vi "svx_Data to Process (DAQmx).vi"(0 "acquisition task":T1={"AI device settings"={"AI DAQmx TaskID"="", "response"=[{"AI physical channel"="Dev1/ai0", "AI channel settings"={"max value [V]"=10.0, "min value [V]"=-10.0, "terminal config"=10083, "DSA channel settings"={"coupling"=10045, "enable IEPE excitation"=FALSE, "IEPE current [mA]"=4.0}}}]}, "acquisition type"=enum."Finite", "measurement settings"={"AI sampling frequency"=51200.0, "AO sampling frequency"=51200.0, "AI block size"=0, "AO block Size"=0, "block duration [ms]"=100.0, "number of AI channels"=0, "device propagation delay [samples]"=0.0, "DUT propagation time [s]"=0.0}, "settling settings"={"settle time"=0.015599999576807022, "settle cycles"=5}, "integration settings"={"integration time"=0.015599999576807022, "integration cycles"=5}, "AO device settings"={"AO DAQmx taskID"="", "excitation"=[]}, "acquisition accounting"={"initial read size [samples]"=0, "read offset [samples]"=0, "read length [samples]"=0, "blocks to settle [samples]"=0, "min delay until transition [samples]"=0}, "frequency range"={"start frequency"=-1.0, "stop frequency"=-1.0}, "block type"=enum."Initialize", "source settings"={"signal type"=enum."Sine wave", "frequency"=0.0, "total amplitude"=0.0, "frequencies"=[1.0], "relative amplitudes"=[1.0], "offset"=1.0, "total amplitude list"=[1.0], "ramping rate"=0.0}, "chirp settings"={"amplitude"=0.0, "frequency range"={"start (Hz)"=20.0, "stop (Hz)"=20000.0, "frequency spacing"=enum."Logarithmic"}, "sampling info"={"Fs"=50000.0, "chirp duration [s]"=3.0}, "initial states"={"frequency [Hz]"=20.0, "phase [rad]"=0.0, "elapsed time [s]"=0.0}, "frequency slope"=0.0, "maximum harmonic"=0, "prefix len [samples]"={"integer"=0, "fractional"=0.0}}} {"chirp settings"."frequency slope" format="%.2f"; "chirp settings"."prefix len [samples]"."fractional" format="%.2p"; "chirp settings"."initial states"."elapsed time [s]" format="%.2f"; "chirp settings"."initial states"."phase [rad]" format="%.2f"; "chirp settings"."initial states"."frequency [Hz]" format="%.2f"; "chirp settings"."sampling info"."chirp duration [s]" format="%.2f"; "chirp settings"."sampling info"."Fs" format="%.2p"; "chirp settings"."frequency range"."stop (Hz)" format="%.2f"; "chirp settings"."frequency range"."start (Hz)" format="%.2f"; "chirp settings"."amplitude" format="%.2f"; "source settings"."total amplitude" format="%.2f"; "source settings"."relative amplitudes" format="%.2f"; "source settings"."frequencies" format="%.2f"; "source settings"."total amplitude list" format="%.2f"; "source settings"."ramping rate" format="%.4f"; "source settings"."offset" format="%.2f"; "source settings"."frequency" format="%.2f"; "frequency range"."stop frequency" format="%.2f"; "frequency range"."start frequency" format="%.2f"; "AO device settings"."excitation"."AO channel settings"."terminal config" items=["Default"=-1, "Differential"=10106, "Pseudodifferential"=12529]; "AI device settings"."response"."AI channel settings"."DSA channel settings"."IEPE current [mA]" min=0.0 max=20.0 format="%.1f"; "AI device settings"."response"."AI channel settings"."DSA channel settings"."coupling" items=["AC"=10045, "DC"=10050, "GND"=10066]; "AI device settings"."response"."AI channel settings"."min value [V]" format="%.2f"; "AI device settings"."response"."AI channel settings"."terminal config" items=["Default"=-1, "RSE"=10083, "NRSE"=10078, "Differential"=10106, "Pseudodifferential"=12529]; "AI device settings"."response"."AI channel settings"."max value [V]" format="%.2f"; "integration settings"."integration time" format="%.2p"; "settling settings"."settle time" format="%.2p"; "measurement settings"."DUT propagation time [s]" format="%.2f"; "measurement settings"."AO sampling frequency" format="%.2f"; "measurement settings"."AI sampling frequency" format="%.2f"}, 5 "waveform data":waveform(dbl)[](array[waveform]), 11 "error in (no error)":errorcluster) -> (4 "acquisition task":T1={"AI device settings"={"AI DAQmx TaskID"="", "response"=[{"AI physical channel"="Dev1/ai0", "AI channel settings"={"max value [V]"=10.0, "min value [V]"=-10.0, "terminal config"=10083, "DSA channel settings"={"coupling"=10045, "enable IEPE excitation"=FALSE, "IEPE current [mA]"=4.0}}}]}, "acquisition type"=enum."Finite", "measurement settings"={"AI sampling frequency"=51200.0, "AO sampling frequency"=51200.0, "AI block size"=0, "AO block Size"=0, "block duration [ms]"=100.0, "number of AI channels"=0, "device propagation delay [samples]"=0.0, "DUT propagation time [s]"=0.0}, "settling settings"={"settle time"=0.015599999576807022, "settle cycles"=5}, "integration settings"={"integration time"=0.015599999576807022, "integration cycles"=5}, "AO device settings"={"AO DAQmx taskID"="", "excitation"=[]}, "acquisition accounting"={"initial read size [samples]"=0, "read offset [samples]"=0, "read length [samples]"=0, "blocks to settle [samples]"=0, "min delay until transition [samples]"=0}, "frequency range"={"start frequency"=-1.0, "stop frequency"=-1.0}, "block type"=enum."Initialize", "source settings"={"signal type"=enum."Sine wave", "frequency"=0.0, "total amplitude"=0.0, "frequencies"=[1.0], "relative amplitudes"=[1.0], "offset"=1.0, "total amplitude list"=[1.0], "ramping rate"=0.0}, "chirp settings"={"amplitude"=0.0, "frequency range"={"start (Hz)"=20.0, "stop (Hz)"=20000.0, "frequency spacing"=enum."Logarithmic"}, "sampling info"={"Fs"=50000.0, "chirp duration [s]"=3.0}, "initial states"={"frequency [Hz]"=20.0, "phase [rad]"=0.0, "elapsed time [s]"=0.0}, "frequency slope"=0.0, "maximum harmonic"=0, "prefix len [samples]"={"integer"=0, "fractional"=0.0}}} {"chirp settings"."frequency slope" format="%.2f"; "chirp settings"."prefix len [samples]"."fractional" format="%.2p"; "chirp settings"."initial states"."elapsed time [s]" format="%.2f"; "chirp settings"."initial states"."phase [rad]" format="%.2f"; "chirp settings"."initial states"."frequency [Hz]" format="%.2f"; "chirp settings"."sampling info"."chirp duration [s]" format="%.2f"; "chirp settings"."sampling info"."Fs" format="%.2p"; "chirp settings"."frequency range"."stop (Hz)" format="%.2f"; "chirp settings"."frequency range"."start (Hz)" format="%.2f"; "chirp settings"."amplitude" format="%.2f"; "source settings"."total amplitude" format="%.2f"; "source settings"."relative amplitudes" format="%.2f"; "source settings"."frequencies" format="%.2f"; "source settings"."total amplitude list" format="%.2f"; "source settings"."ramping rate" format="%.4f"; "source settings"."offset" format="%.2f"; "source settings"."frequency" format="%.2f"; "frequency range"."stop frequency" format="%.2f"; "frequency range"."start frequency" format="%.2f"; "AO device settings"."excitation"."AO channel settings"."terminal config" items=["Default"=-1, "Differential"=10106, "Pseudodifferential"=12529]; "AI device settings"."response"."AI channel settings"."DSA channel settings"."IEPE current [mA]" min=0.0 max=20.0 format="%.1f"; "AI device settings"."response"."AI channel settings"."DSA channel settings"."coupling" items=["AC"=10045, "DC"=10050, "GND"=10066]; "AI device settings"."response"."AI channel settings"."min value [V]" format="%.2f"; "AI device settings"."response"."AI channel settings"."terminal config" items=["Default"=-1, "RSE"=10083, "NRSE"=10078, "Differential"=10106, "Pseudodifferential"=12529]; "AI device settings"."response"."AI channel settings"."max value [V]" format="%.2f"; "integration settings"."integration time" format="%.2p"; "settling settings"."settle time" format="%.2p"; "measurement settings"."DUT propagation time [s]" format="%.2f"; "measurement settings"."AO sampling frequency" format="%.2f"; "measurement settings"."AI sampling frequency" format="%.2f"}, 6 "data to process":waveform(dbl)[](array[waveform]), 8 "new data to process":bool, 15 "error out":errorcluster)   [LabVIEW 2017]
uses:
  <vilib>/addons/Sound and Vibration/Example Support/Audio/DAQmx/svx_Acquisition Task (DAQmx).ctl
  <vilib>/addons/_NISVFA/_Shared subVIs/Controls/svc_Channel Settings.ctl
  <vilib>/addons/_NISVFA/_Shared subVIs/Controls/svc_DSA Channel Settings.ctl
  <vilib>/addons/_NISVFA/_Generation/subVIs/sv_Chirp Settings.ctl
  <vilib>/Waveform/WDTOps.llb/WDT Get Waveform Subset DBL (LV80).vi
  <vilib>/addons/_NISVFA/_Generation/SoundVib_Generation.lvlib
panel:
  in  "empty":waveform(dbl)[](array[waveform])
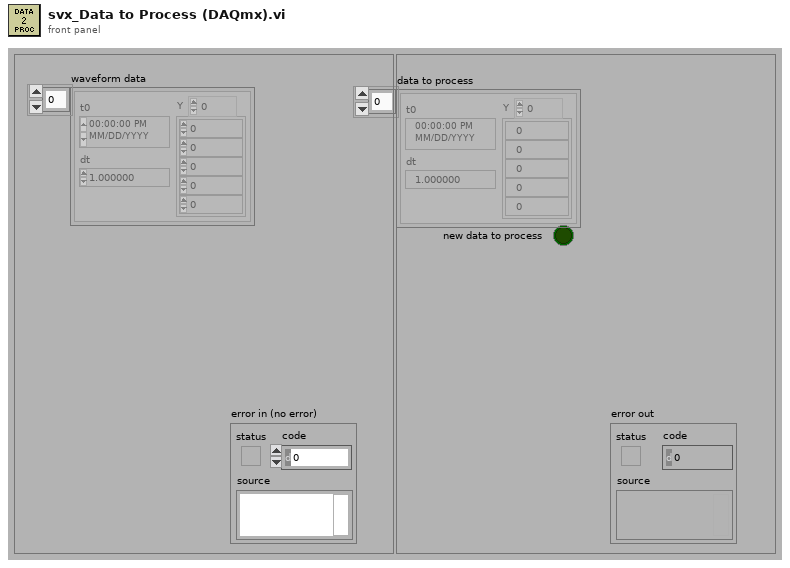
[diagram p1: front panel]
types:
  T1 = typedef "svx_Acquisition Task (DAQmx).ctl" = cluster{"AI device settings":cluster{"AI DAQmx TaskID":refnum<k21>, "response":cluster{"AI physical channel":tag, "AI channel settings":T2}[]}, "acquisition type":enum16{"Finite", "Averaged", "Settled", "Amplitude Sweep", "Stepped Frequency Sweep", "Continuous Frequency Sweep"}, "measurement settings":cluster{"AI sampling frequency":dbl, "AO sampling frequency":dbl, "AI block size":i32, "AO block Size":i32, "block duration [ms]":dbl, "number of AI channels":i32, "device propagation delay [samples]":dbl, "DUT propagation time [s]":dbl}, "settling settings":cluster{"settle time":dbl, "settle cycles":i32}, "integration settings":cluster{"integration time":dbl, "integration cycles":i32}, "AO device settings":cluster{"AO DAQmx taskID":refnum<k21>, "excitation":cluster{"AO physical channel":tag, "AO channel settings":cluster{"maximum value (10 V)":dbl, "minimum value (10 V)":dbl, "terminal config":i32}}[]}, "acquisition accounting":cluster{"initial read size [samples]":i32, "read offset [samples]":i32, "read length [samples]":i32, "blocks to settle [samples]":i32, "min delay until transition [samples]":i32}, "frequency range":cluster{"start frequency":dbl, "stop frequency":dbl}, "block type":enum16{"Initialize", "Settle", "Integrate"}, "source settings":cluster{"signal type":enum16{"Sine wave", "Dual tone (IMD)", "Multitone", "Chirp", "Frequency flat chirp", "Uniform white noise", "Gaussian white noise", "Pink noise", "PRN", "Continuous swept-sine"}, "frequency":dbl, "total amplitude":dbl, "frequencies":dbl[], "relative amplitudes":dbl[], "offset":dbl, "total amplitude list":dbl[], "ramping rate":dbl}, "chirp settings":T4}
  T2 = typedef "svc_Channel Settings.ctl" = cluster{"max value [V]":dbl, "min value [V]":dbl, "terminal config":i32, "DSA channel settings":T3}
  T3 = typedef "svc_DSA Channel Settings.ctl" = cluster{"coupling":i32, "enable IEPE excitation":bool, "IEPE current [mA]":dbl}
  T4 = typedef "SoundVib_Generation.lvlib/sv_Chirp Settings.ctl" = cluster{"amplitude":dbl, "frequency range":cluster{"start (Hz)":dbl, "stop (Hz)":dbl, "frequency spacing":enum16{"Linear", "Logarithmic"}}, "sampling info":cluster{"Fs":dbl, "chirp duration [s]":dbl}, "initial states":cluster{"frequency [Hz]":dbl, "phase [rad]":dbl, "elapsed time [s]":dbl}, "frequency slope":dbl, "maximum harmonic":i32, "prefix len [samples]":cluster{"integer":u32, "fractional":dbl}}
  T5 = enum16{"Finite", "Averaged", "Settled", "Amplitude Sweep", "Stepped Frequency Sweep", "Continuous Frequency Sweep"}
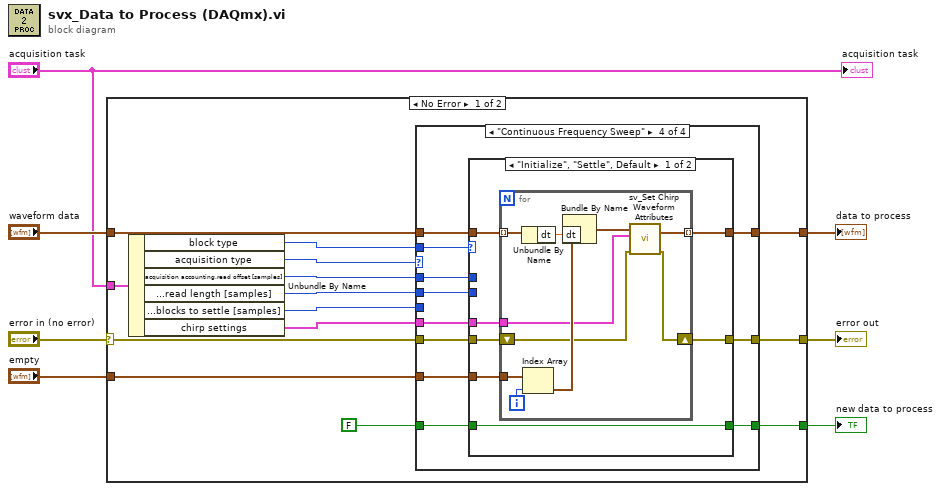
[diagram p0: block diagram]
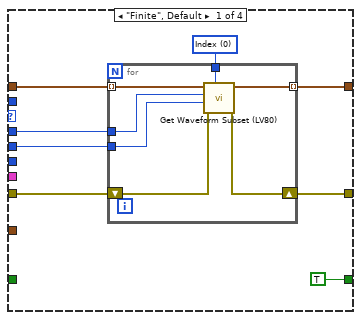
[diagram p2: hidden frame]
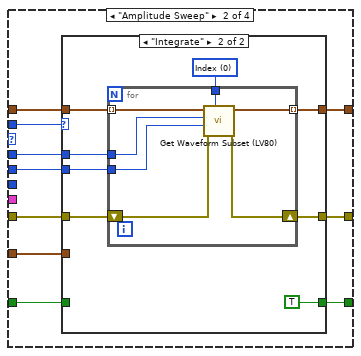
[diagram p3: hidden frame]
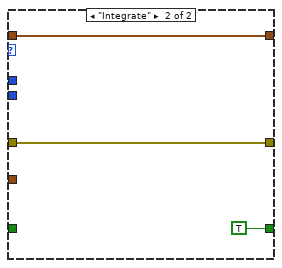
[diagram p6: hidden frame]
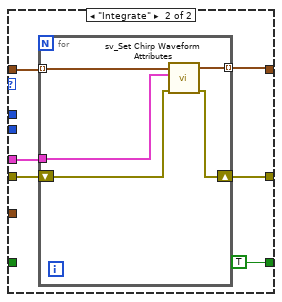
[diagram p7: hidden frame]
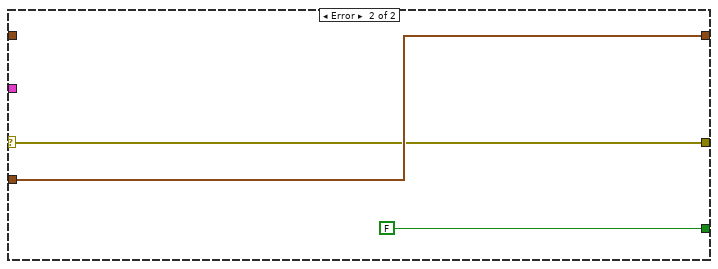
[diagram p8: hidden frame]
diagram:
  n1 = case shown="No Error" "error in (no error)" {
    selector: "error in (no error)" -> [w10 w120]
    tunnel: "acquisition task" -> [w21 _]
    tunnel: [w19 FALSE ("Boolean")] -> w7
    tunnel: "empty" -> [w17 w122]
    tunnel: [w16 w122] -> w5
    tunnel: "waveform data" -> [w15 _]
    tunnel: [w9 w120] -> w2
    frame No Error {
      n2 = Unbundle By Name(w21) -> ("block type"=w20:enum16{"Initialize", "Settle", "Integrate"}, "acquisition type"=w11:T5, "acquisition accounting.read offset [samples]"=w12:i32, "acquisition accounting.read length [samples]"=w13:i32, "acquisition accounting.blocks to settle [samples]"=w14:i32, "chirp settings"=w8:T4)
      n3 = case shown="\"Continuous Frequency Sweep\"" w11 {
        tunnel: w12 -> [w26 w44 w72 w89]
        tunnel: w13 -> [w25 w43 w71 w88]
        tunnel: w14 -> [_ _ _ _]
        tunnel: w15 -> [w29 w46 w74 w91]
        tunnel: [w28 w45 w73 w90] -> w16
        tunnel: w17 -> [_ w42 w70 w87]
        tunnel: FALSE ("Boolean") -> [_ w41 w69 w86]
        tunnel: [TRUE w40 w68 w85] -> w19
        tunnel: w20 -> [_ w39 w67 w84]
        tunnel: w10 -> [w22 w38 w66 w83]
        tunnel: [w23 w37 w65 w82] -> w9
        tunnel: w8 -> [_ _ _ w81]
        frame "Finite", Default {
          w27 = u16 0 items=["Index", "Relative Time"] ("Mode")
          n4 = for {
            tunnel: w29 -> [w36] mode=indexing
            tunnel: w27 -> [w35]
            tunnel: [w34] -> w28 mode=indexing
            tunnel: w26 -> [w33]
            tunnel: w25 -> [w32]
            shift-right: [w31] -> w23
            shift-left: w22 -> [w30]
            n5 = call-poly <vilib>:"Get Waveform Subset (LV80).vi"("start/duration format"=w35, "error in (no error)"=w30, "duration"=w32, "start samples/time"=w33, "waveform in"=w36) -> ("error out"=w31:errorcluster, "waveform out"=w34:waveform(dbl))  [unwired: 1 in, 2 out]
          }
        }
        frame "Amplitude Sweep" {
          n6 = case shown="\"Integrate\"" w39 {
            tunnel: w46 -> [_ w57]
            tunnel: [w49 w56] -> w45
            tunnel: w44 -> [_ w54]
            tunnel: w43 -> [_ w53]
            tunnel: w42 -> [w49 _]
            tunnel: w41 -> [w48 _]
            tunnel: [w48 TRUE] -> w40
            tunnel: w38 -> [w47 w51]
            tunnel: [w47 w50] -> w37
            frame "Initialize", Default {
            }
            frame "Integrate" {
              w55 = u16 0 items=["Index", "Relative Time"] ("Mode")
              n7 = for {
                tunnel: w57 -> [w64] mode=indexing
                tunnel: w55 -> [w63]
                tunnel: [w62] -> w56 mode=indexing
                tunnel: w54 -> [w61]
                tunnel: w53 -> [w60]
                shift-right: [w58] -> w50
                shift-left: w51 -> [w59]
                n8 = call-poly <vilib>:"Get Waveform Subset (LV80).vi"("start/duration format"=w63, "error in (no error)"=w59, "duration"=w60, "start samples/time"=w61, "waveform in"=w64) -> ("error out"=w58:errorcluster, "waveform out"=w62:waveform(dbl))  [unwired: 1 in, 2 out]
              }
            }
          }
        }
        frame "Averaged", "Settled" {
          n9 = case shown="\"Initialize\", \"Settle\", Default" w67 {
            tunnel: w74 -> [_ w78]
            tunnel: [w77 w78] -> w73
            tunnel: w72 -> [_ _]
            tunnel: w71 -> [_ _]
            tunnel: w70 -> [w77 _]
            tunnel: w69 -> [w76 _]
            tunnel: [w76 TRUE] -> w68
            tunnel: w66 -> [w75 w79]
            tunnel: [w75 w79] -> w65
            frame "Initialize", "Settle", Default {
            }
            frame "Integrate" {
            }
          }
        }
        frame "Continuous Frequency Sweep" {
          n10 = case shown="\"Initialize\", \"Settle\", Default" w84 {
            tunnel: w91 -> [w96 w113]
            tunnel: [w94 w112] -> w90
            tunnel: w89 -> [_ _]
            tunnel: w88 -> [_ _]
            tunnel: w87 -> [w97 _]
            tunnel: w86 -> [w98 _]
            tunnel: [w98 TRUE] -> w85
            tunnel: w83 -> [w93 w110]
            tunnel: [w92 w109] -> w82
            tunnel: w81 -> [w95 w111]
            frame "Initialize", "Settle", Default {
              n11 = for {
                tunnel: w97 -> [w108]
                tunnel: w96 -> [w106] mode=indexing
                tunnel: w95 -> [w99]
                tunnel: [w102] -> w94 mode=indexing
                shift-right: [w100] -> w92
                shift-left: w93 -> [w101]
                i -> [w107]
                n12 = Unbundle By Name(w106) -> ("dt"=w105:dbl)
                n13 = Index Array(array=w108, index=w107) -> (element=w104:waveform(dbl))
                n14 = Bundle By Name(cluster=w104, "dt"=w105) -> (w103:waveform(dbl))
                n15 = call <vilib>:"sv_Set Chirp Waveform Attributes.vi"("error in (no error)"=w101, "chirp settings"=w99, "chirp signal"=w103) -> ("error out"=w100:errorcluster, "chirp signal out"=w102:waveform(dbl))  [unwired: 7 in]
              }
            }
            frame "Integrate" {
              n16 = for {
                tunnel: w113 -> [w116] mode=indexing
                tunnel: w111 -> [w115]
                shift-right: [w118] -> w109
                shift-left: w110 -> [w119]
                tunnel: [w117] -> w112 mode=indexing
                n17 = call <vilib>:"sv_Set Chirp Waveform Attributes.vi"("error in (no error)"=w119, "chirp settings"=w115, "chirp signal"=w116) -> ("error out"=w118:errorcluster, "chirp signal out"=w117:waveform(dbl))  [unwired: 7 in]
              }
            }
          }
        }
      }
    }
    frame Error {
    }
  }
  "new data to process" <- w7
  "data to process" <- w5
  "error out" <- w2
  "acquisition task" <- "acquisition task"
